vi "Range Mask.vi"() -> ()   [LabVIEW 2016]
panel:
  out "Range":u32 format="%x"
  in  "Address":u32 format="%.0x"
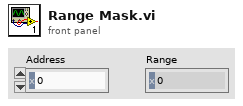
[diagram p1: front panel]
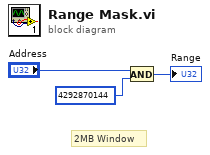
[diagram p0: block diagram]
diagram:
  # "2MB Window"
  n1 = And(x="Address", y=u32 4292870144) -> (x .and. y?=→"Range":u32)
